vi "Test Error Propagation Lunit Verify File.vi"(8 "error in":errorcluster, 11 "Error.Tests in":refnum<class "Error.Propagation.Tests.lvclass">) -> (0 "error out":errorcluster, 3 "Error.Tests out":refnum<class "Error.Propagation.Tests.lvclass">)   [LabVIEW 2020, in "Error.Propagation.Tests.lvclass"]
uses:
  Error.Propagation.Tests.lvclass
  Source/Approval Tests/Options/Options.lvclass
  <vilib>/Astemes/LUnit/Test Case.lvclass
  <vilib>/addons/_JKI Toolkits/Caraya/classes/Assert/Assert True.vi
  <vilib>/addons/_JKI Toolkits/Caraya/classes/Assert/Assert Equal Value and Type_Variant.vi
  <vilib>/addons/_JKI Toolkits/Caraya/classes/Test/Test.lvclass
  <vilib>/addons/_JKI Toolkits/Caraya/classes/Assert/Assert.lvclass
  Source/Extensions/LUnit.Extension/LUnit.Extension.lvlib
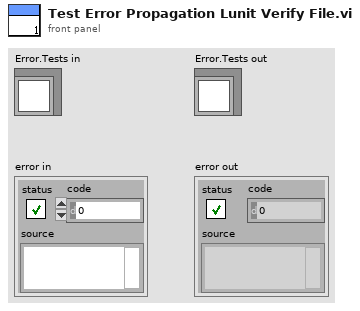
[diagram p1: front panel]
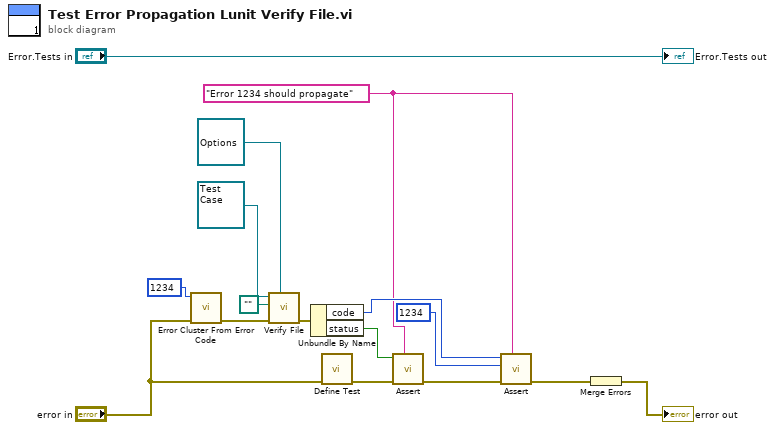
[diagram p0: block diagram]
diagram:
  w2 = "Error 1234 should propagate" ("Label (VI Title)")
  n1 = call <vilib>:"Error Cluster From Error Code.vi"("error in (no error)"="error in", "error code (0)"=1234) -> ("error out"=w13:errorcluster)  [unwired: 7 in]
  n2 = call "Verify File.vi"("Options"=refnum<class "Options.lvclass"> refnum, "error in"=w13, "path to file"=path "", "LUnit Test Case In"=refnum<class "Test Case.lvclass"> refnum) -> ("error out"=w12:errorcluster)  [unwired: 6 in, 1 out]
  n3 = Unbundle By Name(w12) -> ("code"=w4:i32, "status"=w5:bool)
  n4 = call <vilib>:"Define Test.vi"("error in (no error)"="error in") -> ("error out"=w16:errorcluster)  [unwired: 9 in, 1 out]
  n5 = call-poly <vilib>:"Assert.vi"("Label"=w2, "error in (no error)"=w16, "True?"=w5) -> ("error out"=w11:errorcluster)  [unwired: 7 in, 1 out]
  n6 = call-poly <vilib>:"Assert.vi"("Label"=w2, "error in (no error)"=w11, "Actual"=1234 ("error code (1)"), "Expected"=w4) -> ("error out"=w10:errorcluster)  [unwired: 6 in, 1 out]
  n7 = Merge Errors(w10) -> (→"error out":errorcluster)
  "Error.Tests out" <- "Error.Tests in"
